vi "Create Shortcut.vi"(8 "error in (no error)":errorcluster, 10 "Arguments":T1={"Description"="Shortcut generated by LabVIEW", "Hotkey"="", "IconLocation"="%SystemRoot%\\system32\\SHELL32.dll, 41", "RelativePath"="", "TargetPath"="%SystemRoot%\\notepad.exe", "WindowStyle"=1, "WorkingDirectory"="C:\\Documents and Settings\\All Users\\Desktop", "Arguments"=[]} {"WindowStyle" items=["Restore"=1, "Maximized"=3, "Minimized"=7]}, 11 "PathLink":string="C:\\Documents and Settings\\All Users\\Desktop\\MyNewShortcut.lnk") -> (0 "error out":errorcluster)   [LabVIEW 2010]
panel:
  # "By Troy Kujawski"
  # "PathLink: String value indicating the pathname of the shortcut to create.\nDescription: property contains a string value describing a shortcut.\nFullName: property contains a string value indicating the fully qualified path to the shortcut's target.\nHotkey: A string representing the key-combination to assign to the shortcut.\nIconLocation: Assigns an icon to a shortcut, or identifies the icon assigned to a shortcut.\nRelativePath: Assigns a relative path to a shortcut, or identifies the relative path of a shortcut.\nTargetPath: The path to the shortcut's executable.\nWindowStyle: Assigns a window style to a shortcut, or identifies the type of window style used by a shortcut.\nWorkingDirectory: Assign a working directory to a shortcut, or identifies the working directory used by a shortcut."
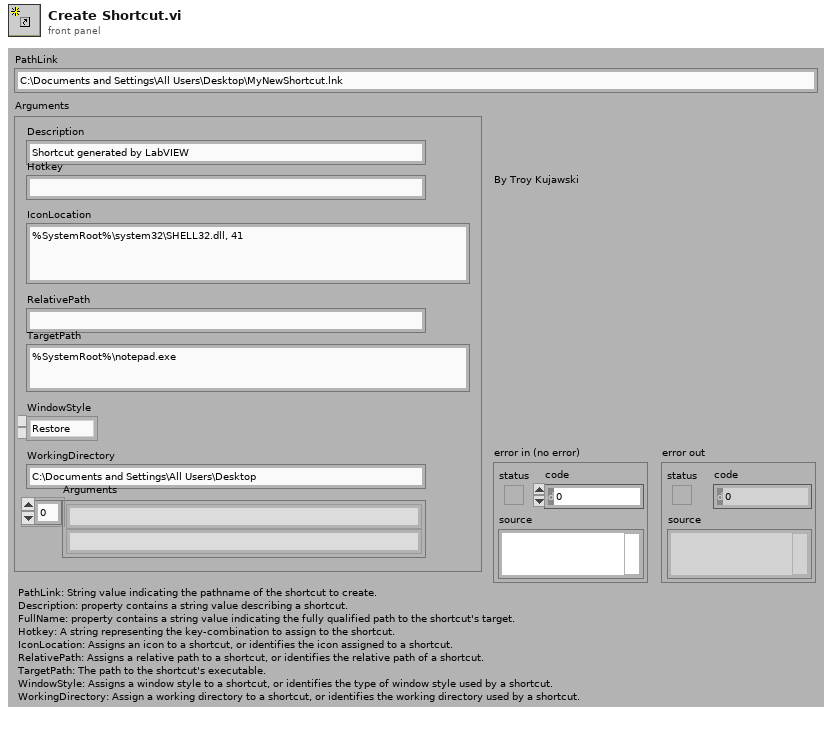
[diagram p1: front panel]
types:
  T1 = cluster{"Description":string, "Hotkey":string, "IconLocation":string, "RelativePath":string, "TargetPath":string, "WindowStyle":i32, "WorkingDirectory":string, "Arguments":string[]}
  T2 = enum16{"Description", "Hotkey", "IconLocation", "RelativePath", "TargetPath", "WindowStyle", "WorkingDirectory", "Arguments"}[]
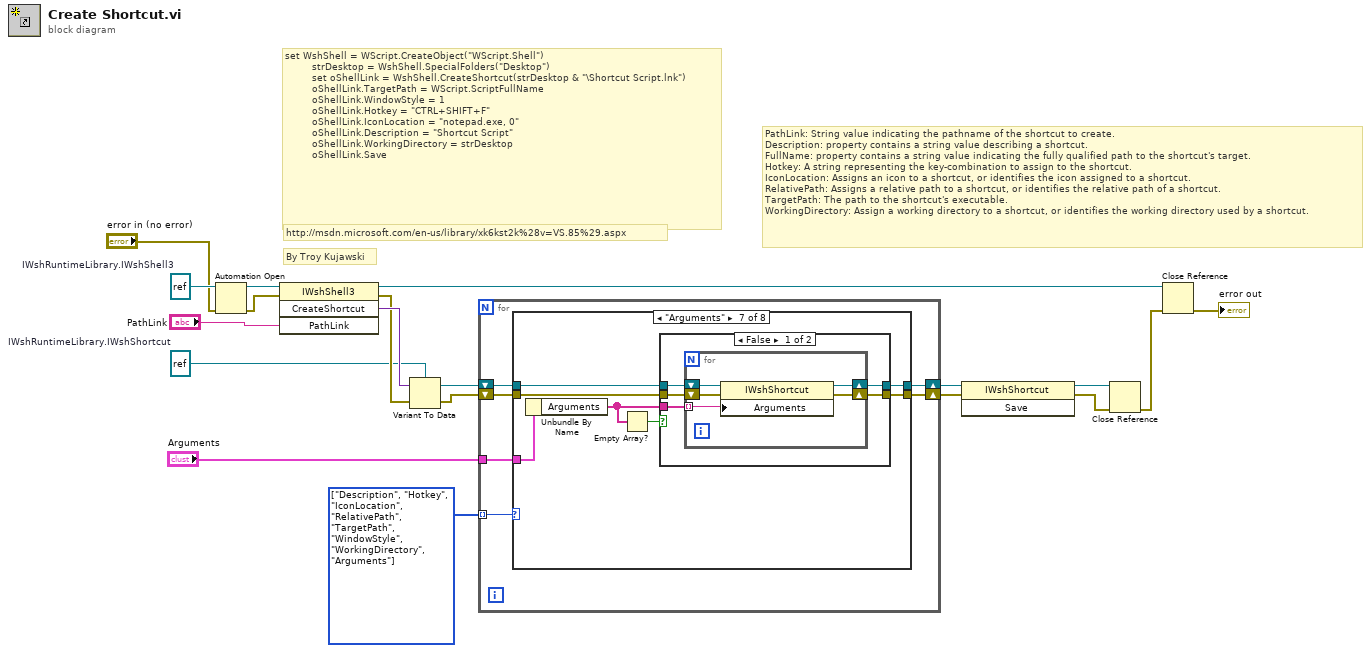
[diagram p0: block diagram]
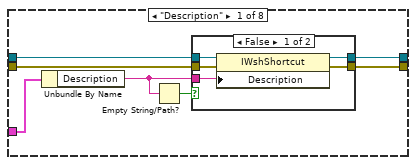
[diagram p2: hidden frame]
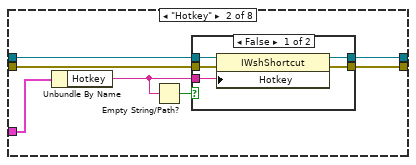
[diagram p4: hidden frame]
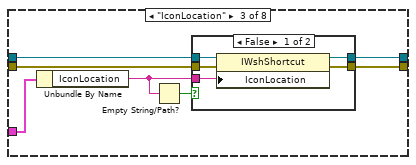
[diagram p6: hidden frame]
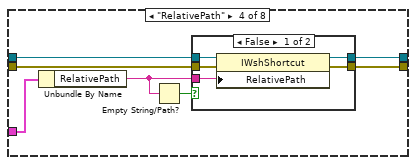
[diagram p8: hidden frame]
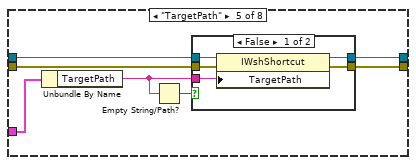
[diagram p10: hidden frame]
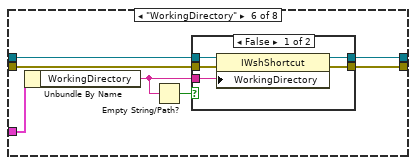
[diagram p12: hidden frame]
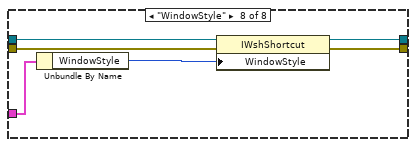
[diagram p15: hidden frame]
diagram:
  w3 = T2 [enum."Description", enum."Hotkey", enum."IconLocation", enum."RelativePath", enum."TargetPath", enum."WindowStyle", enum."WorkingDirectory", enum."Arguments"] items=["Description", "Hotkey", "IconLocation", "RelativePath", "TargetPath", "WindowStyle", "WorkingDirectory", "Arguments"]
  w19 = refnum<k7> refnum  # IWshRuntimeLibrary.IWshShell3
  w6 = refnum<k7> refnum  # IWshRuntimeLibrary.IWshShortcut
  # "By Troy Kujawski"
  # "PathLink: String value indicating the pathname of the shortcut to create.\nDescription: property contains a string value describing a shortcut.\nFullName: property contains a string value indicating the fully qualified path to the shortcut's target.\nHotkey: A string representing the key-combination to assign to the shortcut.\nIconLocation: Assigns an icon to a shortcut, or identifies the icon assigned to a shortcut.\nRelativePath: Assigns a relative path to a shortcut, or identifies the relative path of a shortcut.\nTargetPath: The path to the shortcut's executable.\nWorkingDirectory: Assign a working directory to a shortcut, or identifies the working directory used by a shortcut."
  # "http://msdn.microsoft.com/en-us/library/xk6kst2k%28v=VS.85%29.aspx"
  # "set WshShell = WScript.CreateObject(\"WScript.Shell\")\n         strDesktop = WshShell.SpecialFolders(\"Desktop\")\n         set oShellLink = WshShell.CreateShortcut(strDesktop & \"\\Shortcut Script.lnk\")\n         oShellLink.TargetPath = WScript.ScriptFullName\n         oShellLink.WindowStyle = 1\n         oShellLink.Hotkey = \"CTRL+SHIFT+F\"\n         oShellLink.IconLocation = \"notepad.exe, 0\"\n         oShellLink.Description = \"Shortcut Script\"\n         oShellLink.WorkingDirectory = strDesktop\n         oShellLink.Save"
  n1 = Automation Open(error in (no error)="error in (no error)", Automation Refnum=w19) -> (Automation Refnum=w18:refnum<k7>, error out=w17:errorcluster)  [unwired: 2 in]
  n2 = invoke class="IWshShell3" method="CreateShortcut"(reference=w18, error in=w17, "PathLink"="PathLink") -> (reference out=w16:refnum<k7>, error out=w14:errorcluster, "CreateShortcut"=w15:variant)  [unwired: 1 in, 1 out]
  n3 = Variant To Data(error in=w14, Variant=w15, type=w6) -> (error out=w12:errorcluster, data=w13:refnum<k7>)
  n4 = for {
    tunnel: "Arguments" -> [w21]
    shift-right: [w23] -> w10
    shift-left: w13 -> [w25]
    shift-right: [w22] -> w8
    shift-left: w12 -> [w24]
    tunnel: w3 -> [w20] mode=indexing
    n5 = case shown="\"Arguments\"" w20 {
      tunnel: w25 -> [w32 w46 w60 w74 w88 w102 w116 w134]
      tunnel: w24 -> [w31 w45 w59 w73 w87 w101 w115 w133]
      tunnel: [w30 w44 w58 w72 w86 w100 w114 w132] -> w23
      tunnel: [w29 w43 w57 w71 w85 w99 w113 w131] -> w22
      tunnel: w21 -> [w28 w42 w56 w70 w84 w98 w112 w130]
      frame "Description" {
        n6 = Unbundle By Name(w28) -> ("Description"=w27:string)
        n7 = Empty String/Path?(string/path=w27) -> (empty?=w26:bool)
        n8 = case shown="False" w26 {
          tunnel: w32 -> [w37 w39]
          tunnel: w31 -> [w36 w38]
          tunnel: [w35 w39] -> w30
          tunnel: [w34 w38] -> w29
          tunnel: w27 -> [w33 _]
          frame False {
            n9 = property class="IWshShortcut"(reference=w37, error in=w36, "Description"=w33) -> (reference out=w35:refnum<k7>, error out=w34:errorcluster)
          }
          frame True {
          }
        }
      }
      frame "Hotkey" {
        n10 = Unbundle By Name(w42) -> ("Hotkey"=w41:string)
        n11 = Empty String/Path?(string/path=w41) -> (empty?=w40:bool)
        n12 = case shown="False" w40 {
          tunnel: w46 -> [w51 w53]
          tunnel: w45 -> [w50 w52]
          tunnel: [w49 w53] -> w44
          tunnel: [w48 w52] -> w43
          tunnel: w41 -> [w47 _]
          frame False {
            n13 = property class="IWshShortcut"(reference=w51, error in=w50, "Hotkey"=w47) -> (reference out=w49:refnum<k7>, error out=w48:errorcluster)
          }
          frame True {
          }
        }
      }
      frame "IconLocation" {
        n14 = Unbundle By Name(w56) -> ("IconLocation"=w55:string)
        n15 = Empty String/Path?(string/path=w55) -> (empty?=w54:bool)
        n16 = case shown="False" w54 {
          tunnel: w60 -> [w65 w67]
          tunnel: w59 -> [w64 w66]
          tunnel: [w63 w67] -> w58
          tunnel: [w62 w66] -> w57
          tunnel: w55 -> [w61 _]
          frame False {
            n17 = property class="IWshShortcut"(reference=w65, error in=w64, "IconLocation"=w61) -> (reference out=w63:refnum<k7>, error out=w62:errorcluster)
          }
          frame True {
          }
        }
      }
      frame "RelativePath" {
        n18 = Unbundle By Name(w70) -> ("RelativePath"=w69:string)
        n19 = Empty String/Path?(string/path=w69) -> (empty?=w68:bool)
        n20 = case shown="False" w68 {
          tunnel: w74 -> [w79 w81]
          tunnel: w73 -> [w78 w80]
          tunnel: [w77 w81] -> w72
          tunnel: [w76 w80] -> w71
          tunnel: w69 -> [w75 _]
          frame False {
            n21 = property class="IWshShortcut"(reference=w79, error in=w78, "RelativePath"=w75) -> (reference out=w77:refnum<k7>, error out=w76:errorcluster)
          }
          frame True {
          }
        }
      }
      frame "TargetPath" {
        n22 = Unbundle By Name(w84) -> ("TargetPath"=w83:string)
        n23 = Empty String/Path?(string/path=w83) -> (empty?=w82:bool)
        n24 = case shown="False" w82 {
          tunnel: w88 -> [w93 w95]
          tunnel: w87 -> [w92 w94]
          tunnel: [w91 w95] -> w86
          tunnel: [w90 w94] -> w85
          tunnel: w83 -> [w89 _]
          frame False {
            n25 = property class="IWshShortcut"(reference=w93, error in=w92, "TargetPath"=w89) -> (reference out=w91:refnum<k7>, error out=w90:errorcluster)
          }
          frame True {
          }
        }
      }
      frame "WorkingDirectory" {
        n26 = Unbundle By Name(w98) -> ("WorkingDirectory"=w97:string)
        n27 = Empty String/Path?(string/path=w97) -> (empty?=w96:bool)
        n28 = case shown="False" w96 {
          tunnel: w102 -> [w107 w109]
          tunnel: w101 -> [w106 w108]
          tunnel: [w105 w109] -> w100
          tunnel: [w104 w108] -> w99
          tunnel: w97 -> [w103 _]
          frame False {
            n29 = property class="IWshShortcut"(reference=w107, error in=w106, "WorkingDirectory"=w103) -> (reference out=w105:refnum<k7>, error out=w104:errorcluster)
          }
          frame True {
          }
        }
      }
      frame "Arguments" {
        n30 = Unbundle By Name(w112) -> ("Arguments"=w111:string[])
        n31 = Empty Array?(array=w111) -> (empty?=w110:bool)
        n32 = case shown="False" w110 {
          tunnel: w116 -> [w121 w128]
          tunnel: w115 -> [w120 w127]
          tunnel: [w119 w128] -> w114
          tunnel: [w118 w127] -> w113
          tunnel: w111 -> [w117 _]
          frame False {
            n33 = for {
              tunnel: w117 -> [w122] mode=indexing
              shift-right: [w124] -> w119
              shift-left: w121 -> [w126]
              shift-right: [w123] -> w118
              shift-left: w120 -> [w125]
              n34 = property class="IWshShortcut"(reference=w126, error in=w125, "Arguments"=w122) -> (reference out=w124:refnum<k7>, error out=w123:errorcluster)
            }
          }
          frame True {
          }
        }
      }
      frame "WindowStyle" {
        n35 = Unbundle By Name(w130) -> ("WindowStyle"=w129:i32)
        n36 = property class="IWshShortcut"(reference=w134, error in=w133, "WindowStyle"=w129) -> (reference out=w132:refnum<k7>, error out=w131:errorcluster)
      }
    }
  }
  n37 = invoke class="IWshShortcut" method="Save"(reference=w10, error in=w8) -> (reference out=w9:refnum<k7>, error out=w7:errorcluster)  [unwired: 1 in, 1 out]
  n38 = Close Reference(reference=w9, error in (no error)=w7) -> (error out=w11:errorcluster)
  n39 = Close Reference(reference=w16, error in (no error)=w11) -> (error out=→"error out":errorcluster)
